vi "Initialize Network.vi"(8 "error in (no error)":errorcluster, 10 "RDB References":T4 {"RDB Send Reference"."RDB Data"."payload" format="%x"; "RDB Send Reference"."RDB Data"."timestamp" format="%<%.7X\n%x>T"; "RDB Send Reference"."RDB Data"."type" items=["FlexRay Data"=32, "FlexRay Null"=33, "FlexRay Symbol"=34, "Log Trigger"=225, "Start Trigger"=226]; "RDB Send Reference"."RDB Data"."cycle count" max=63 step=1; "RDB Receive Reference"."RDB Data"."payload" format="%x"; "RDB Receive Reference"."RDB Data"."timestamp" format="%<%.7X\n%x>T"; "RDB Receive Reference"."RDB Data"."type" items=["FlexRay Data"=32, "FlexRay Null"=33, "FlexRay Symbol"=34, "Log Trigger"=225, "Start Trigger"=226]; "RDB Receive Reference"."RDB Data"."cycle count" max=63 step=1}, 11 "Settings":T1={"UDP Receiver"=refnum, "UDP Sender"=refnum, "Valid Packet"=FALSE, "TCP"=refnum, "Network Settings"={"IP adress"="127.0.0.1", "RDB"={"Protocol"=enum."UDP", "Tx Port"=48270, "Rx Port"=10, "Buffer Size"=204800, "Timeout"=10}, "SCP"={"Protocol"=enum."TCP", "Tx Port"=48191, "Rx Port"=48191, "Buffer Size"=204800, "Timeout"=10}}, "vclient"=path ""}) -> (0 "error out":errorcluster, 2 "RDB References":T4 {"RDB Send Reference"."RDB Data"."payload" format="%x"; "RDB Send Reference"."RDB Data"."timestamp" format="%<%.7X\n%x>T"; "RDB Send Reference"."RDB Data"."type" items=["FlexRay Data"=32, "FlexRay Null"=33, "FlexRay Symbol"=34, "Log Trigger"=225, "Start Trigger"=226]; "RDB Send Reference"."RDB Data"."cycle count" max=63 step=1; "RDB Receive Reference"."RDB Data"."payload" format="%x"; "RDB Receive Reference"."RDB Data"."timestamp" format="%<%.7X\n%x>T"; "RDB Receive Reference"."RDB Data"."type" items=["FlexRay Data"=32, "FlexRay Null"=33, "FlexRay Symbol"=34, "Log Trigger"=225, "Start Trigger"=226]; "RDB Receive Reference"."RDB Data"."cycle count" max=63 step=1}, 3 "Settings":T1={"UDP Receiver"=refnum, "UDP Sender"=refnum, "Valid Packet"=FALSE, "TCP"=refnum, "Network Settings"={"IP adress"="127.0.0.1", "RDB"={"Protocol"=enum."UDP", "Tx Port"=48270, "Rx Port"=10, "Buffer Size"=204800, "Timeout"=10}, "SCP"={"Protocol"=enum."TCP", "Tx Port"=48191, "Rx Port"=48191, "Buffer Size"=204800, "Timeout"=10}}, "vclient"=path ""})   [LabVIEW 2020, in "Vires VTD Engine.lvlib"]
uses:
  Vires VTD Engine.lvlib
  Type/Settings.ctl
  Shared/Network Settings.ctl
  Shared/Protocol.ctl
  RDB/RDB References.ctl
  RDB/RDB Reference.ctl
  <vilib>/xnet/xnet.llb/XNET Frame FlexRay.ctl
  <vilib>/xnet/xnet.llb/XNET Frame Type FlexRay.ctl
  Shared/Vires VTD Shared.lvlib
  RDB/RDB.lvlib
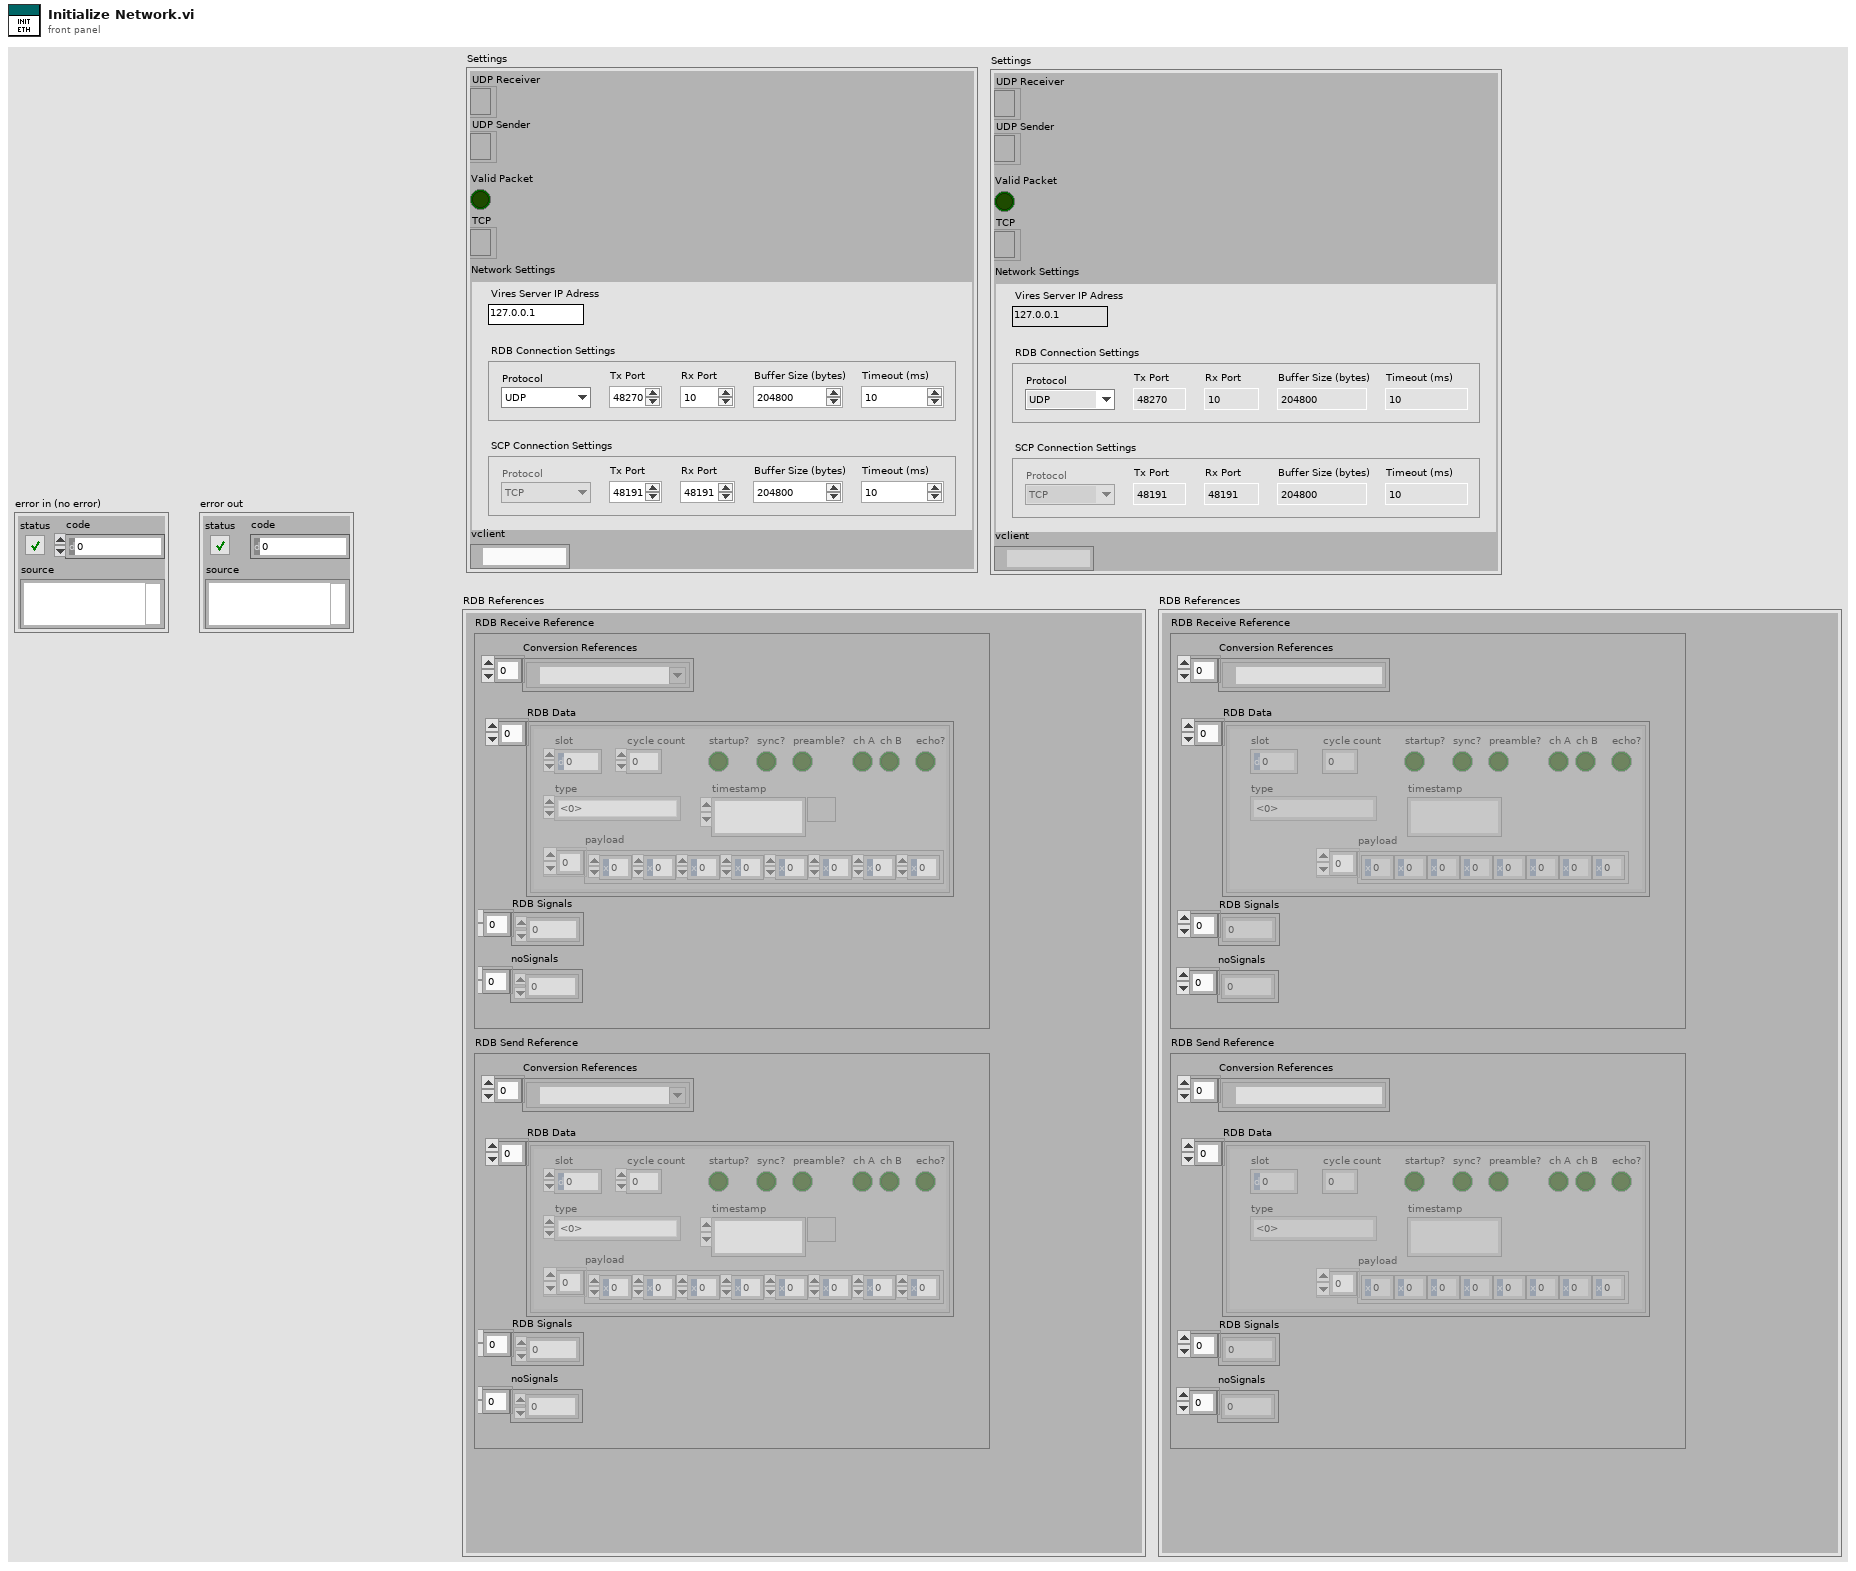
[diagram p1: front panel]
types:
  T1 = typedef "Vires VTD Engine.lvlib/Settings.ctl" = cluster{"UDP Receiver":refnum<k16>, "UDP Sender":refnum<k16>, "Valid Packet":bool, "TCP":refnum<k5>, "Network Settings":T2, "vclient":path}
  T2 = typedef "Vires VTD Shared.lvlib/Network Settings.ctl" = cluster{"IP adress":string, "RDB":cluster{"Protocol":T3, "Tx Port":u16, "Rx Port":u16, "Buffer Size":i32, "Timeout":u16}, "SCP":cluster{"Protocol":T3, "Tx Port":u16, "Rx Port":u16, "Buffer Size":i32, "Timeout":u16}}
  T3 = typedef "Vires VTD Shared.lvlib/Protocol.ctl" = enum16{"UDP", "TCP"}
  T4 = typedef "RDB.lvlib/RDB References.ctl" = cluster{"RDB Receive Reference":T5, "RDB Send Reference":T5}
  T5 = typedef "RDB.lvlib/RDB Reference.ctl" = cluster{"Conversion References":refnum<k21>[], "RDB Data":T6[], "RDB Signals":dbl[], "noSignals":i32[]}
  T6 = typedef "XNET Frame FlexRay.ctl" = cluster{"timestamp":timestamp, "payload":u8[], "slot":u16, "type":T7, "cycle count":u8, "startup?":bool, "sync?":bool, "preamble?":bool, "ch A":bool, "ch B":bool, "echo?":bool}
  T7 = typedef "XNET Frame Type FlexRay.ctl" = u8
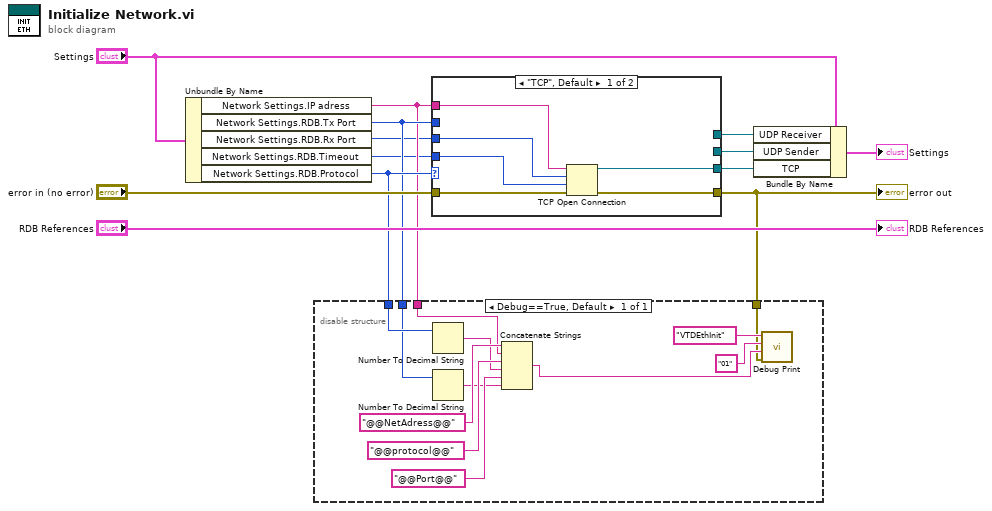
[diagram p0: block diagram]
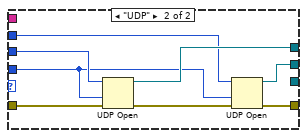
[diagram p2: hidden frame]
diagram:
  n1 = Unbundle By Name("Settings") -> ("Network Settings.IP adress"=w4:string, "Network Settings.RDB.Tx Port"=w5:u16, "Network Settings.RDB.Rx Port"=w2:u16, "Network Settings.RDB.Timeout"=w1:u16, "Network Settings.RDB.Protocol"=w6:T3)
  n2 = case shown="\"TCP\", Default" w6 {
    tunnel: "error in (no error)" -> [w19 w27]
    tunnel: [w18 w25] -> w7
    tunnel: [_ w24] -> w12
    tunnel: [w17 _] -> w10
    tunnel: [_ w23] -> w9
    tunnel: w4 -> [w16 _]
    tunnel: w5 -> [_ w22]
    tunnel: w2 -> [w14 w21]
    tunnel: w1 -> [w15 w20]
    frame "TCP", Default {
      n3 = TCP Open Connection(address=w16, remote port or service name=w14, timeout ms (60000)=w15, error in (no error)=w19) -> (connection ID=w17:refnum<k5>, error out=w18:errorcluster)  [unwired: 1 in]
    }
    frame "UDP" {
      n4 = UDP Open(8:w27, 9:w20, 11:w21) -> (port=w23:refnum<k16>, 0:w26:errorcluster)  [unwired: 2 in, 1 out]
      n5 = UDP Open(8:w26, 9:w20, 11:w22) -> (port=w24:refnum<k16>, 0:w25:errorcluster)  [unwired: 2 in, 1 out]
    }
  }
  "error out" <- w7
  n6 = disable-structure shown="Debug==True, Default" {
    disable-tunnel: w5 -> [w28]
    disable-tunnel: w6 -> [w29]
    disable-tunnel: w4 -> [w31]
    disable-tunnel: w7 -> [w30]
    frame condition #0 (active) {
      n7 = Number To Decimal String(number=w29) -> (decimal integer string=w36:string)  [unwired: 1 in]
      n8 = Number To Decimal String(number=w28) -> (decimal integer string=w34:string)  [unwired: 1 in]
      n9 = Concatenate Strings("@@NetAdress@@" ("string"), w31, "@@protocol@@" ("string"), w36, "@@Port@@" ("string"), w34) -> (w33:string)
      n10 = call "Debug Print.vi"("error out"=w30, "comment"=w33, "Index"="01", "Module"="VTDEthInit") -> ()  [unwired: 8 in]
    }
  }
  n11 = Bundle By Name(cluster="Settings", "UDP Receiver"=w9, "UDP Sender"=w12, "TCP"=w10) -> (→"Settings":T1)
  "RDB References" <- "RDB References"
